vi "Export settings_Core.vi"(10 "2D Array of Names Values IN":string[][](array[string]), 11 "Controls[]":refnum<vi>[](array[refnum])) -> (2 "2D Array of Names Values OUT":string[][](array[string]))   [LabVIEW 2011]
uses:
  <vilib>/Utility/VariantDataType/VariantType.lvlib
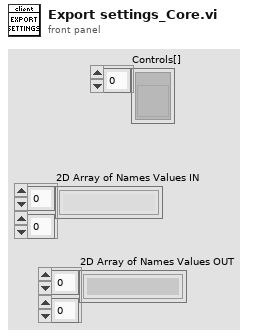
[diagram p1: front panel]
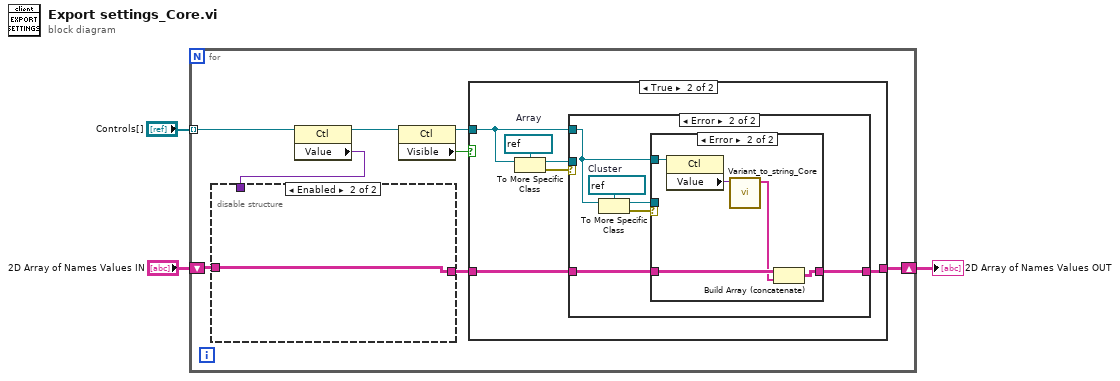
[diagram p0: block diagram]
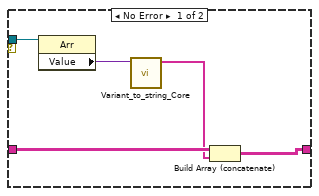
[diagram p3: hidden frame]
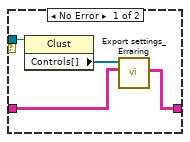
[diagram p4: hidden frame]
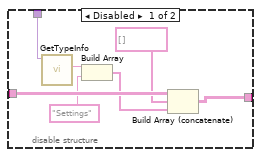
[diagram p5: hidden frame]
diagram:
  n1 = for {
    tunnel: "Controls[]" -> [w9] mode=indexing
    shift-right: [w10] -> w1
    shift-left: "2D Array of Names Values IN" -> [w11]
    n2 = property on="Property Node" class="Ctl"(reference=w9) -> (reference out=w6:refnum<vi>, "Value"=w8:variant)  [unwired: 1 in, 1 out]
    n3 = disable-structure shown="Enabled" {
      disable-tunnel: w11 -> [w45 w46]
      disable-tunnel: w8 -> [w44 _]
      disable-tunnel: [w43 w46] -> w7
      frame Disabled {
        n4 = call <vilib>:"GetTypeInfo.vi"("Variant"=w44) -> ("Name"=w42:string)  [unwired: 6 in, 4 out]
        n5 = Build Array(w42, "Settings" ("element")) -> (w40:string[])
        n6 = Build Array (concatenate)(w45, string[] [] ("appended array"), w40) -> (w43:string[][])
      }
      frame Enabled {
      }
    }
    n7 = property on="Property Node" class="Ctl"(reference=w6) -> (reference out=w5:refnum<vi>, "Visible"=w4:bool)  [unwired: 1 in, 1 out]
    n8 = case shown="True" w4 {
      tunnel: [w12 w18] -> w10
      tunnel: w7 -> [w12 w17]
      tunnel: w5 -> [_ w13]
      frame False {
      }
      frame True {
        w16 = refnum<vi> refnum  # Array
        n9 = To More Specific Class(target class=w16, reference=w13) -> (specific class reference=w14:refnum<vi>, error out=w15:errorcluster)  [unwired: 1 in]
        n10 = case shown="Error" w15 {
          tunnel: w14 -> [w23 _]
          tunnel: w13 -> [_ w28]
          tunnel: [w19 w25] -> w18
          tunnel: w17 -> [w21 w24]
          frame No Error {
            n11 = property class="Arr"(reference=w23) -> ("Value"=w22:variant)  [unwired: 1 in, 2 out]
            n12 = call "Variant_to_string_Core.vi"("Value"=w22) -> ("1D_Array_String_Setting_Name_Value"=w20:string[])  [unwired: 10 in]
            n13 = Build Array (concatenate)(w21, w20) -> (w19:string[][])
          }
          frame Error {
            w29 = refnum<vi> refnum  # Cluster
            n14 = To More Specific Class(target class=w29, reference=w28) -> (specific class reference=w26:refnum<vi>, error out=w27:errorcluster)  [unwired: 1 in]
            n15 = case shown="Error" w27 {
              tunnel: w28 -> [_ w37]
              tunnel: w26 -> [w33 _]
              tunnel: [w30 w34] -> w25
              tunnel: w24 -> [w31 w36]
              frame No Error {
                n16 = property on="Property Node" class="Clust"(reference=w33) -> ("Controls[]"=w32:refnum<vi>[])  [unwired: 1 in, 2 out]
                n17 = call "Export settings_Erraring.vi"("2D Array of Names Values IN"=w31, "Controls[]"=w32) -> ("2D Array of Names Values OUT"=w30:string[][])  [unwired: 9 in]
              }
              frame Error {
                n18 = property on="Property Node" class="Ctl"(reference=w37) -> ("Value"=w38:variant)  [unwired: 1 in, 2 out]
                n19 = call "Variant_to_string_Core.vi"("Value"=w38) -> ("1D_Array_String_Setting_Name_Value"=w35:string[])  [unwired: 10 in]
                n20 = Build Array (concatenate)(w36, w35) -> (w34:string[][])
              }
            }
          }
        }
      }
    }
  }
  "2D Array of Names Values OUT" <- w1
